vi "Configure Trigger.vi"(0 "VISA resource name":refnum<visa-resource-name>, 5 "error in (no error)":errorcluster, 6 "Source (0: Immediate)":u16(ring) items=["Immediate", "Bus", "External"], 7 "Auto Delay? (T: Auto)":bool=TRUE, 8 "Sample Count (1)":i32=1 min=1 max=50000, 9 "Trigger Delay (0.0015 s)":dbl=0.0015 min=0.0 max=3600.0 format="%#.6g", 10 "Trigger Count (1)":i32=1 min=1 max=50000) -> (14 "VISA resource name out":refnum<visa-resource-name>, 19 "error out":errorcluster)   [LabVIEW 2020, in "Keithley 2100 Series.lvlib"]
doc: "This VI configures the trigger settings on the instrument."
uses:
  Keithley 2100 Series.lvlib
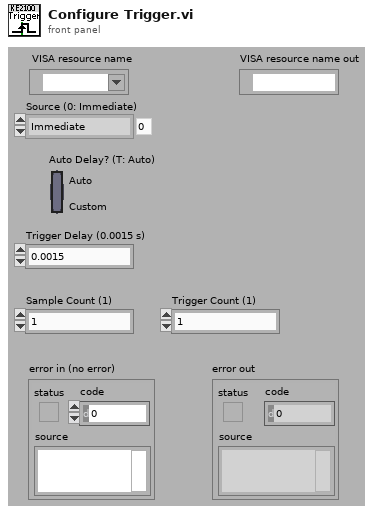
[diagram p1: front panel]
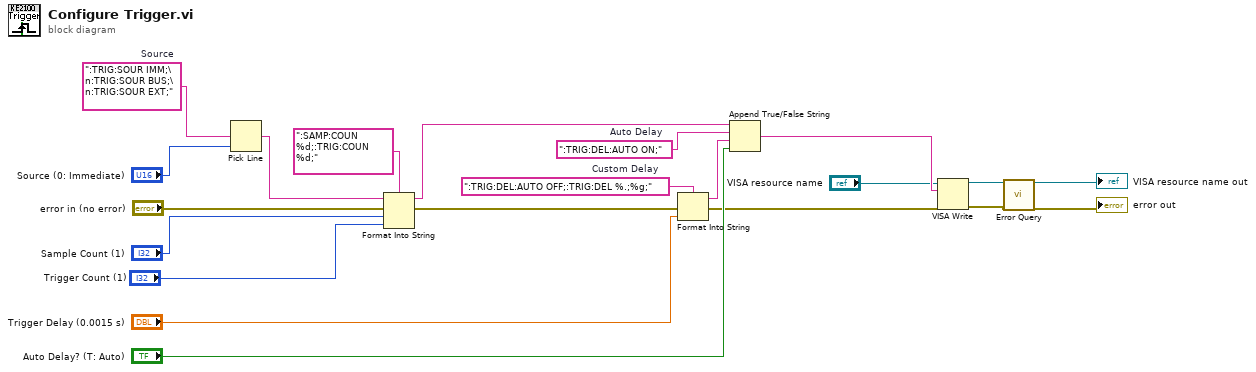
[diagram p0: block diagram]
diagram:
  w18 = ":TRIG:DEL:AUTO ON;"  # Auto Delay
  w20 = ":TRIG:DEL:AUTO OFF;:TRIG:DEL %.;%g;"  # Custom Delay
  w14 = ":TRIG:SOUR IMM;\n:TRIG:SOUR BUS;\n:TRIG:SOUR EXT;"  # Source
  n1 = Pick Line(multi-line string=w14, line index="Source (0: Immediate)") -> (output string=w9:string)  [unwired: 1 in]
  n2 = Format Into String(format string=":SAMP:COUN %d;:TRIG:COUN %d;", initial string=w9, error in="error in (no error)", "Sample Count (1)", "Trigger Count (1)") -> (resulting string=w8:string, error out=w10:errorcluster)
  n3 = Format Into String(format string=w20, error in=w10, "Trigger Delay (0.0015 s)") -> (resulting string=w19:string, error out=w12:errorcluster)  [unwired: 1 in]
  n4 = Append True/False String(1:"Auto Delay? (T: Auto)", 2:w19, 3:w18, 4:w8) -> (0:w16:string)
  n5 = VISA Write(VISA resource name="VISA resource name", write buffer=w16, error in (no error)=w12) -> (VISA resource name out=w4:refnum<visa-resource-name>, error out=w3:errorcluster)  [unwired: 1 out]
  n6 = call "Error Query.vi"("VISA resource name"=w4, "error in (no error)"=w3) -> ("VISA resource name out"=→"VISA resource name out":refnum<visa-resource-name>, "error out"=→"error out":errorcluster)  [unwired: 14 in, 2 out]
